vi "Get Source Preference.vi"(8 "error in (no error)":errorcluster, 11 "VISA resource name":refnum<visa-resource-name>) -> (0 "error out":errorcluster, 2 "Source Preference":i32, 3 "VISA resource name out":refnum<visa-resource-name>)   [LabVIEW 2014, in "Fluke 5XXX Series Multicalibrators.lvlib"]
doc: "This VI return the source preference from 5500A Calibrator or 5725A Amplifier, when a 5725A Amplifier is attached.\n\nNote:\n\nThis VI is available only for instrument model 5500A."
uses:
  Fluke 5XXX Series Multicalibrators.lvlib
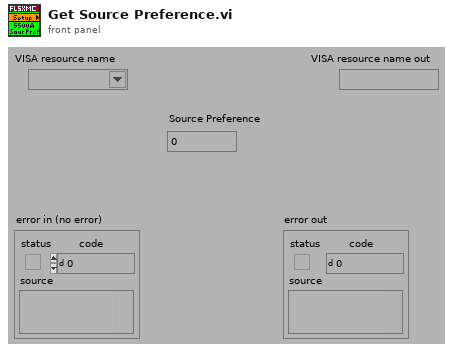
[diagram p1: front panel]
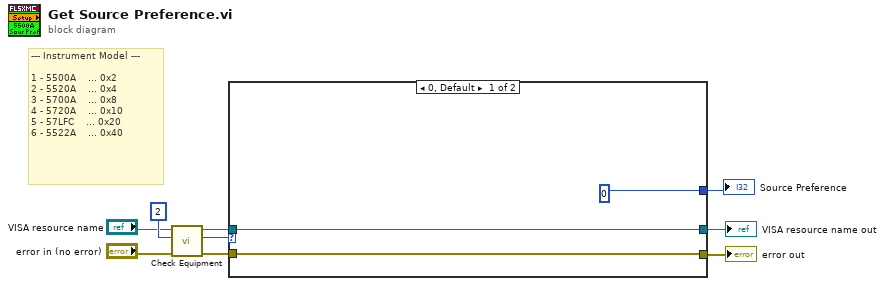
[diagram p0: block diagram]
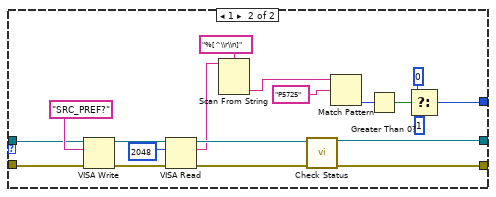
[diagram p2: hidden frame]
diagram:
  # "--- Instrument Model ---\n\n1 - 5500A    ... 0x2\n2 - 5520A    ... 0x4\n3 - 5700A    ... 0x8\n4 - 5720A    ... 0x10\n5 - 57LFC    ... 0x20\n6 - 5522A    ... 0x40"
  n1 = call "Check Equipment.vi"("error in (no error)"="error in (no error)", "Bit Mask"=2 ("Numeric"), "VISA resource name"="VISA resource name") -> ("error out"=w9:errorcluster, "Present?"=w8:u32, "VISA resource name out"=w7:refnum<visa-resource-name>)  [unwired: 6 in]
  n2 = case shown="0, Default" w8 {
    tunnel: [w11 w25] -> w3
    tunnel: [w10 w22] -> w2
    tunnel: w9 -> [w11 w27]
    tunnel: w7 -> [w10 w26]
    tunnel: [0 w13] -> w1
    frame 0, Default {
    }
    frame 1 {
      n3 = VISA Write(VISA resource name=w26, write buffer="SRC_PREF?", error in (no error)=w27) -> (VISA resource name out=w30:refnum<visa-resource-name>, error out=w29:errorcluster)  [unwired: 1 out]
      n4 = VISA Read(VISA resource name=w30, byte count=u32 2048 ("byte count (0)"), error in (no error)=w29) -> (VISA resource name out=w23:refnum<visa-resource-name>, read buffer=w15:string, error out=w24:errorcluster)  [unwired: 1 out]
      n5 = Scan From String(format string="%[^\\r\\n]", input string=w15) -> (output 1=w14:string)  [unwired: 3 in, 3 out]
      n6 = call "Check Status.vi"("VISA resource name"=w23, "error in (no error)"=w24) -> ("VISA resource name out"=w22:refnum<visa-resource-name>, "error out"=w25:errorcluster)  [unwired: 12 in]
      n7 = Match Pattern(string=w14, regular expression="P5725") -> (offset past match=w19:i32)  [unwired: 1 in, 3 out]
      n8 = Greater Than 0?(x=w19) -> (x > 0?=w16:bool)
      n9 = Select(t=u16 0 ("f"), s=w16, f=u16 1) -> (s? t:f=w13:u16)
    }
  }
  "Source Preference" <- w1
  "VISA resource name out" <- w2
  "error out" <- w3
